vi "Compile and Export Settings.vi"(8 "error in (no error)":errorcluster, 11 "Device Item Ref in":T1 format="%.0x") -> (0 "error out":errorcluster)   [LabVIEW 2023, in "Protection and Counter Addon System Explorer.lvlib"]
uses:
  Protection and Counter Addon System Explorer.lvlib
  <vilib>/NI VeriStand/Custom Device API/Custom Device Item Ref.ctl
  Addon Shared/Types/Exported.OnCompile.ctl
  Addon Shared/Types/XNET Settings.ctl
  SubModules/Frame-Protection-Support/Source/Shared/Types/Exported Frame Settings.ctl
  SubModules/Frame-Protection-Support/Source/Shared/Types/Exported Frame Type.ctl
  SubModules/Frame-Protection-Support/Source/Shared/Types/Exported Protection Settings.ctl
  SubModules/Frame-Protection-Support/Source/Shared/Types/Protection Type.ctl
  SubModules/Frame-Protection-Support/Source/Shared/Types/XNET Signal Configuration.ctl
  SubModules/Frame-Protection-Support/Source/Shared/Types/Exported Counter Settings.ctl
  SubModules/Frame-Protection-Support/Source/Shared/Types/Exported Event Trigger Type.ctl
  Addon Shared/Types/986x.ctl
  SubModules/Frame-Protection-Support/Source/System Explorer/Types/Export Frame GUIDs List.ctl
  <vilib>/NI VeriStand/Custom Device Tools/Custom Device Utility Library/Search Direction.ctl
  SubModules/Frame-Protection-Support/Source/System Explorer/Types/Export Frames List and Type.ctl
  SubModules/Frame-Protection-Support/Source/System Explorer/Types/Exported Frame Settings.ctl
  Addon Shared/SubVIs/GUID Lookup.vi
  <vilib>/NI VeriStand/Custom Device API/NI VeriStand - Get Item Property.vi
  <vilib>/NI VeriStand/Custom Device API/Get Item Property (Boolean).vi
  <vilib>/NI VeriStand/Custom Device API/Get Item Property (String).vi
  FileDependency.Get.Target Path.vi
  <vilib>/NI VeriStand/Custom Device Tools/Custom Device Utility Library/NI VeriStand - Search for Item by GUID.vi
  <vilib>/NI VeriStand/Custom Device API/Set Item Property (Variant).vi
  <vilib>/NI VeriStand/Custom Device Tools/Custom Device Utility Library/Custom Device Utility Library.lvlib
  Addon Shared/Protection and Counter Addon Shared.lvlib
  <vilib>/NI VeriStand/Custom Device API/Custom Device API.lvlib
  SubModules/Frame-Protection-Support/Source/Shared/Protection and Counter Support Shared.lvlib
  <vilib>/NI/NIVS Inline Async API/_Data Access System Explorer/Data Access System Explorer.lvlib
  SubModules/Frame-Protection-Support/Source/System Explorer/Protection and Counter Support System Explorer.lvlib
  SubModules/Frame-Protection-Support/Source/LP_CRC/LP_CRC.lvlib
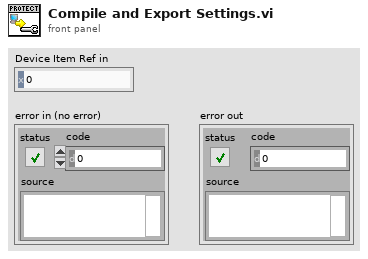
[diagram p1: front panel]
types:
  T1 = typedef "Custom Device API.lvlib/Custom Device Item Ref.ctl" = u64
  T2 = cluster{"Name":string, "Type":enum16{"Output/Write", "Input/Read", "Input/ReadWrite"}, "VS Refs":T1[]}
  T3 = typedef "Protection and Counter Support System Explorer.lvlib/Export Frames List and Type.ctl" = cluster{"Type":T4, "Frame Refs":T1[], "Frame Settings":T5[]}
  T4 = typedef "Protection and Counter Support Shared.lvlib/Exported Frame Type.ctl" = enum16{"Periodic", "Event", "Periodic/Event"}
  T5 = typedef "Protection and Counter Support System Explorer.lvlib/Exported Frame Settings.ctl" = cluster{"ID":u32, "Disable Transmission":bool, "Disable Transmission Ref":T1, "Transmit Trigger":T6, "Transmit Trigger Ref":T1, "Start Time Offset (ms)":u32}
  T6 = typedef "Protection and Counter Support Shared.lvlib/Exported Event Trigger Type.ctl" = enum16{"Channel value change", "Trigger channel (not zero)", "Channel value change or trigger channel (not zero)", "Trigger channel (any value change)", "Channel value change or trigger channel (any value change)"}
  T7 = typedef "Custom Device Utility Library.lvlib/Search Direction.ctl" = enum16{"Down", "Up"}
  T8 = typedef "Protection and Counter Support System Explorer.lvlib/Export Frame GUIDs List.ctl" = cluster{"Signal Page GUID":string, "Rolling Counter Value GUID":string, "Protection Value GUID":string, "Time Difference GUID":string, "Receive Time GUID":string}
  T9 = typedef "Protection and Counter Addon Shared.lvlib/Exported.OnCompile.ctl" = cluster{"Name":string, "XNET Settings":T10, "Frames":T11[], "986x Support":T16, "Incoming Frames":T11[], "Msg IDs":string[], "Data IDs":string[]}
  T10 = typedef "Protection and Counter Addon Shared.lvlib/XNET Settings.ctl" = cluster{"Database":refnum<k21>, "Cluster":refnum<k21>, "Port":string, "Baud rate [Bd]":u64, "Termination":u32, "CAN I/O Mode":u32, "FD Baud rate [Bd]":u64, "Priority":i32, "Use Legacy":bool, "FD ISO Mode":u32}
  T11 = typedef "Protection and Counter Support Shared.lvlib/Exported Frame Settings.ctl" = cluster{"Type":T4, "Frame ID":u32, "Payload Length":u32, "Signal XNET Paths":string[], "Frame.PrevData":dbl[], "VS Offset":i32, "VS Length":i32, "Generation Period":u32, "Has Protection?":bool, "Protection Configurations":T12[], "Has Counter":bool, "Counter Configurations":T15[], "Has Disable?":bool, "Disable VS Index":i32, "Transmit Trigger":T6, "Trigger VS Index":i32, "Start Time Offset (ms)":u32}
  T12 = typedef "Protection and Counter Support Shared.lvlib/Exported Protection Settings.ctl" = cluster{"Protection Frame Index":i32, "Protection Type":T13, "Data Indeces":i32[], "Initialized Data Array":dbl[], "Protection Signal XNET Paths":string[], "CRC Channels":T14[], "Protection VS Update Index":i32, "Override Index":i32, "Override Value Index":i32}
  T13 = typedef "Protection and Counter Support Shared.lvlib/Protection Type.ctl" = enum16{"Arb ID + Bytes Checksum with Inversion", "Arb ID + Bytes CRC with Inversion", "Reversed Raw Signal Checksum with Inversion", "Concatenated Two's Compliment", "LP_CRC8", "LP_Checksum", "LP_CRC8_MRS"}
  T14 = typedef "Protection and Counter Support Shared.lvlib/XNET Signal Configuration.ctl" = cluster{"Start Bit":i32, "Name":string, "Number of bits":i32, "Scale":dbl, "Offset":dbl, "Data Type":u32, "Counter":bool}
  T15 = typedef "Protection and Counter Support Shared.lvlib/Exported Counter Settings.ctl" = cluster{"Frame Index":i32, "Max Count":dbl, "VS Index":i32, "Bit Length":i64, "Override Index":i32, "Override Value Index":i32}
  T16 = typedef "Protection and Counter Addon Shared.lvlib/986x.ctl" = cluster{"Enable":bool, "RIO Device":string, "Bitfile":path}
  T17 = typedef "Custom Device API.lvlib/Custom Device Item Info.ctl" = cluster{"Name":string, "Is Channel":bool, "GUID":string, "Is Waveform":bool}
  T18 = typedef "Protection and Counter Addon System Explorer.lvlib/Frame Settings.ctl" = cluster{"ID":u32, "Disable Transmission":bool, "Disable Transmission Ref":T1, "Transmit Trigger":T19, "Transmit Trigger Ref":T1, "Start Time Offset (ms)":u32}
  T19 = typedef "Protection and Counter Addon System Explorer.lvlib/Event Trigger Type.ctl" = enum16{"Channel value change", "Trigger channel (not zero)", "Channel value change or trigger channel (not zero)", "Trigger channel (any value change)", "Channel value change or trigger channel (any value change)"}
  T20 = cluster{"Name":string, "Type":enum16{"Output/Write", "Input/Read", "Input/ReadWrite"}, "VS Refs":T1[]}[]
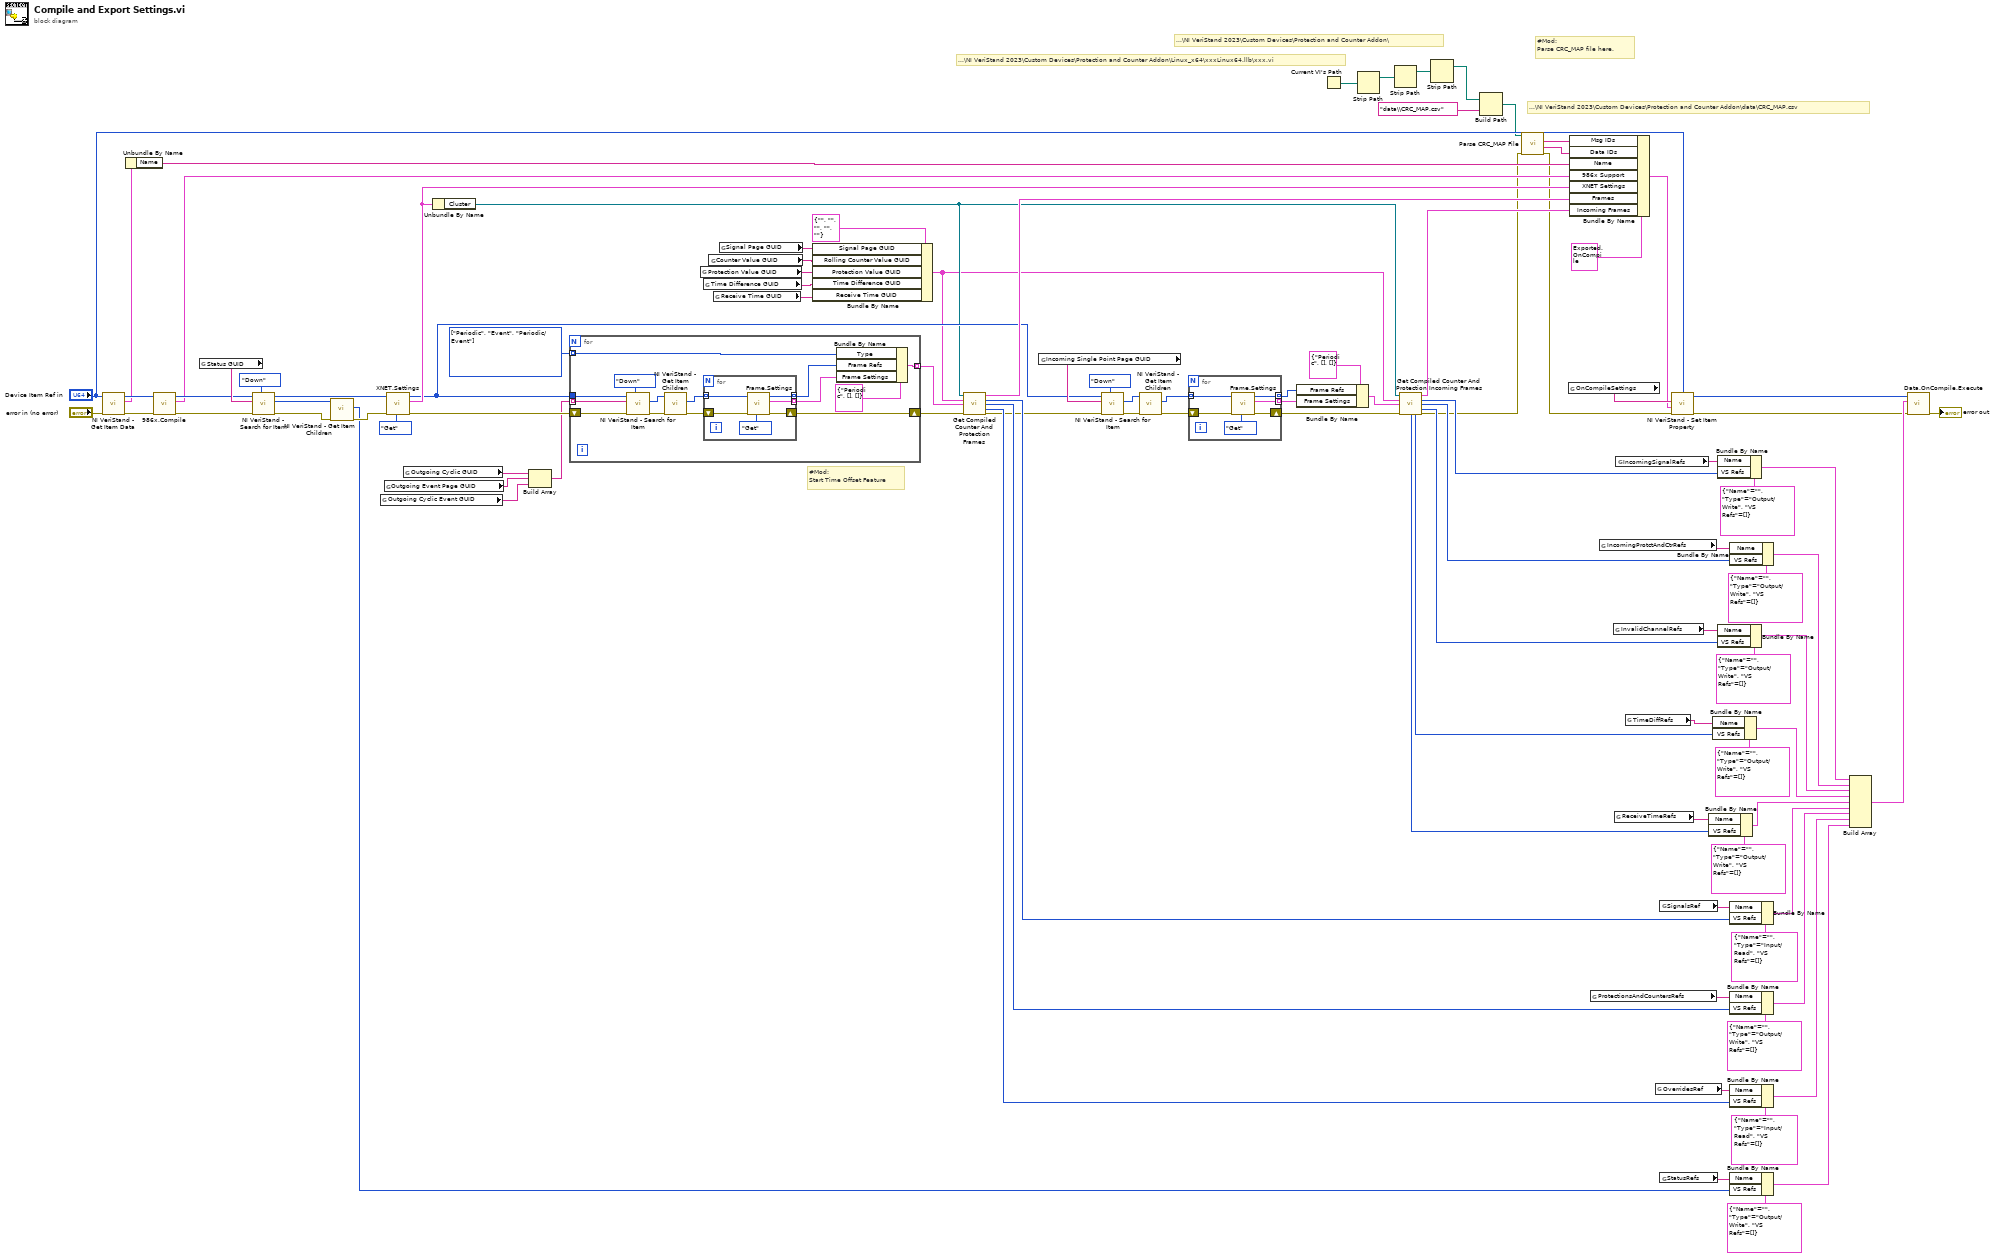
[diagram p0: block diagram]
diagram:
  w70 = T4[] [enum."Periodic", enum."Event", enum."Periodic/Event"] items=["Periodic", "Event", "Periodic/Event"]
  # "#Mod:\nParse CRC_MAP file here."
  # "...\\NI VeriStand 2023\\Custom Devices\\Protection and Counter Addon\\data\\CRC_MAP.csv"
  # "...\\NI VeriStand 2023\\Custom Devices\\Protection and Counter Addon\\"
  # "...\\NI VeriStand 2023\\Custom Devices\\Protection and Counter Addon\\Linux_x64\\xxxLinux64.llb\\xxx.vi"
  # "#Mod:\nStart Time Offset Feature"
  n1 = call <vilib>:"NI VeriStand - Get Item Data.vi"("error in (no error)"="error in (no error)", "Item Ref in"="Device Item Ref in") -> ("error out"=w57:errorcluster, "Item Info"=w55:T17, "Item Ref out"=w56:T1)  [unwired: 6 in, 1 out]
  n2 = Unbundle By Name(w55) -> ("Name"=w54:string)
  n3 = call "986x.Compile.vi"("error in (no error)"=w57, "Item Ref in"=w56) -> ("error out"=w77:errorcluster, "986x Support"=w67:T16, "Item Ref out"=w76:T1)  [unwired: 7 in]
  n4 = global read "GUID Lookup.vi" "Status GUID"() -> (w84:string)
  n5 = call-poly <vilib>:"NI VeriStand - Search for Item.vi"("Direction (Down)"=Search_Direction."Down", "error in"=w77, "Item GUID"=w84, "Section Ref in"=w76) -> ("error out"=w81:errorcluster, "Item Ref"=w82:T1, "Section Ref out"=w83:T1)  [unwired: 4 in, 1 out]
  n6 = call <vilib>:"NI VeriStand - Get Item Children.vi"("error in (no error)"=w81, "Item Ref in"=w82) -> ("error out"=w80:errorcluster, "Child Refs"=w79:T1[])  [unwired: 6 in, 2 out]
  n7 = global read "GUID Lookup.vi" "Outgoing Cyclic Event GUID"() -> (w62:string)
  n8 = global read "GUID Lookup.vi" "Outgoing Event Page GUID"() -> (w63:string)
  n9 = call "XNET.Settings.vi"("Action"=enum8{"Get", "Set"}."Get", "error in (no error)"=w80, "Parent Ref in"=w83) -> ("error out"=w61:errorcluster, "XNET Settings"=w99:T10, "Item Ref out"=w41:T1)  [unwired: 6 in]
  n10 = global read "GUID Lookup.vi" "Outgoing Cyclic GUID"() -> (w64:string)
  n11 = Unbundle By Name(w99) -> ("Cluster"=w25:refnum<k21>)
  n12 = Build Array(w64, w63, w62) -> (w60:string[])
  n13 = for {
    shift-right: [w102] -> w71
    shift-left: w61 -> [w112]
    tunnel: w70 -> [w115] mode=indexing
    tunnel: [w114] -> w69 mode=indexing
    tunnel: w41 -> [w111]
    tunnel: w60 -> [w110] mode=indexing
    n14 = call-poly <vilib>:"NI VeriStand - Search for Item.vi"("Direction (Down)"=Search_Direction."Down", "error in"=w112, "Item GUID"=w110, "Section Ref in"=w111) -> ("error out"=w108:errorcluster, "Item Ref"=w109:T1)  [unwired: 4 in, 2 out]
    n15 = call <vilib>:"NI VeriStand - Get Item Children.vi"("error in (no error)"=w108, "Item Ref in"=w109) -> ("error out"=w106:errorcluster, "Child Refs"=w105:T1[])  [unwired: 6 in, 2 out]
    n16 = for {
      tunnel: w105 -> [w119] mode=indexing
      shift-right: [w118] -> w102
      shift-left: w106 -> [w120]
      tunnel: [w117] -> w104 mode=indexing
      tunnel: [w116] -> w103 mode=indexing
      n17 = call "Frame.Settings.vi"("Action"=enum8{"Get", "Set"}."Get", "error in (no error)"=w120, "Item Ref in"=w119) -> ("error out"=w118:errorcluster, "Frame.Settings"=w116:T18, "Item Ref out"=w117:T1)  [unwired: 6 in]
    }
    n18 = Bundle By Name(cluster=T3 {"Type"=enum."Periodic", "Frame Refs"=[], "Frame Settings"=[]} ("Export Frames List and Type"), "Type"=w115, "Frame Refs"=w104, "Frame Settings"=w103) -> (w114:T3)
  }
  n19 = global read "GUID Lookup.vi" "Protection Value GUID"() -> (w73:string)
  n20 = global read "GUID Lookup.vi" "Time Difference GUID"() -> (w12:string)
  n21 = global read "GUID Lookup.vi" "Counter Value GUID"() -> (w74:string)
  n22 = global read "GUID Lookup.vi" "Receive Time GUID"() -> (w11:string)
  n23 = global read "GUID Lookup.vi" "Signal Page GUID"() -> (w75:string)
  n24 = Bundle By Name(cluster=T8 {"Signal Page GUID"="", "Rolling Counter Value GUID"="", "Protection Value GUID"="", "Time Difference GUID"="", "Receive Time GUID"=""}, "Signal Page GUID"=w75, "Rolling Counter Value GUID"=w74, "Protection Value GUID"=w73, "Time Difference GUID"=w12, "Receive Time GUID"=w11) -> (w24:T8)
  n25 = call "Get Compiled Counter And Protection Frames.vi"("XNET Cluster"=w25, "GUIDs"=w24, "Frames per type"=w69, "error in (no error)"=w71) -> ("Frames"=w65:T11[], "Signals Refs"=w66:T1[], "Counters and Protection Refs"=w94:T1[], "Override Refs"=w50:T1[], "error out"=w46:errorcluster)  [unwired: 7 in]
  n26 = global read "GUID Lookup.vi" "Incoming Single Point Page GUID"() -> (w45:string)
  n27 = call-poly <vilib>:"NI VeriStand - Search for Item.vi"("Direction (Down)"=Search_Direction."Down", "error in"=w46, "Item GUID"=w45, "Section Ref in"=w41) -> ("error out"=w47:errorcluster, "Item Ref"=w48:T1)  [unwired: 4 in, 2 out]
  n28 = call <vilib>:"NI VeriStand - Get Item Children.vi"("error in (no error)"=w47, "Item Ref in"=w48) -> ("error out"=w44:errorcluster, "Child Refs"=w42:T1[])  [unwired: 6 in, 2 out]
  n29 = for {
    tunnel: w42 -> [w125] mode=indexing
    shift-right: [w124] -> w43
    shift-left: w44 -> [w126]
    tunnel: [w123] -> w39 mode=indexing
    tunnel: [w122] -> w38 mode=indexing
    n30 = call "Frame.Settings.vi"("Action"=enum8{"Get", "Set"}."Get", "error in (no error)"=w126, "Item Ref in"=w125) -> ("error out"=w124:errorcluster, "Frame.Settings"=w122:T18, "Item Ref out"=w123:T1)  [unwired: 6 in]
  }
  n31 = Bundle By Name(cluster=T3 {"Type"=enum."Periodic", "Frame Refs"=[], "Frame Settings"=[]} ("Export Frames List and Type"), "Frame Refs"=w39, "Frame Settings"=w38) -> (w23:T3)
  n32 = Current VI's Path() -> (path=w10:path)
  n33 = Strip Path(path=w10) -> (stripped path=w9:path)  [unwired: 1 out]
  n34 = Strip Path(path=w9) -> (stripped path=w8:path)  [unwired: 1 out]
  n35 = call "Get Compiled Counter And Protection Incoming Frames.vi"("XNET Cluster"=w25, "GUIDs"=w24, "Incoming Frames In"=w23, "error in (no error)"=w43) -> ("Incoming Frames Out"=w22:T11[], "Signals Refs"=w21:T1[], "Counters and Protection Refs"=w20:T1[], "Invalid Refs"=w19:T1[], "Rcv Time Refs"=w17:T1[], "Time Diff Refs"=w18:T1[], "error out"=w2:errorcluster)  [unwired: 5 in]
  n36 = Strip Path(path=w8) -> (stripped path=w7:path)  [unwired: 1 out]
  n37 = Build Path(base path=w7, name or relative path="data\\CRC_MAP.csv") -> (appended path=w3:path)
  n38 = call "Parse CRC_MAP File.vi"("error in"=w2, "file (use dialog)"=w3) -> ("error out"=w1:errorcluster, "Data IDs"=w4:string[], "Msg IDs"=w5:string[])  [unwired: 6 in, 1 out]
  n39 = global read "GUID Lookup.vi" "OnCompileSettings"() -> (w89:string)
  n40 = Bundle By Name(cluster=T9 {"Name"="", "XNET Settings"={"Database"="", "Cluster"="", "Port"="", "Baud rate [Bd]"=500000, "Termination"=1, "CAN I/O Mode"=0, "FD Baud rate [Bd]"=500000, "Priority"=100, "Use Legacy"=FALSE, "FD ISO Mode"=0}, "Frames"=[], "986x Support"={"Enable"=FALSE, "RIO Device"="", "Bitfile"=path ""}, "Incoming Frames"=[], "Msg IDs"=[], "Data IDs"=[]}, "Msg IDs"=w5, "Data IDs"=w4, "Name"=w54, "986x Support"=w67, "XNET Settings"=w99, "Frames"=w65, "Incoming Frames"=w22) -> (w30:T9)
  n41 = global read "GUID Lookup.vi" "ProtectionsAndCountersRefs"() -> (w90:string)
  n42 = global read "GUID Lookup.vi" "IncomingProtctAndCtrRefs"() -> (w26:string)
  n43 = global read "GUID Lookup.vi" "InvalidChannelRefs"() -> (w34:string)
  n44 = global read "GUID Lookup.vi" "ReceiveTimeRefs"() -> (w33:string)
  n45 = global read "GUID Lookup.vi" "IncomingSignalRefs"() -> (w35:string)
  n46 = global read "GUID Lookup.vi" "TimeDiffRefs"() -> (w29:string)
  n47 = global read "GUID Lookup.vi" "OverridesRef"() -> (w53:string)
  n48 = global read "GUID Lookup.vi" "SignalsRef"() -> (w91:string)
  n49 = global read "GUID Lookup.vi" "StatusRefs"() -> (w86:string)
  n50 = call-poly <vilib>:"NI VeriStand - Set Item Property.vi"("error in (no error)"=w1, "Value"=w30, "Property Name"=w89, "Item Ref in"="Device Item Ref in") -> ("error out"=w93:errorcluster, "Item Ref out"=w92:T1)  [unwired: 5 in, 1 out]
  n51 = Bundle By Name(cluster=T2 {"Name"="", "Type"=enum."Output/Write", "VS Refs"=[]} ("Group"), "Name"=w33, "VS Refs"=w17) -> (w13:T2)
  n52 = Bundle By Name(cluster=T2 {"Name"="", "Type"=enum."Output/Write", "VS Refs"=[]} ("Group"), "Name"=w29, "VS Refs"=w18) -> (w14:T2)
  n53 = Bundle By Name(cluster=T2 {"Name"="", "Type"=enum."Output/Write", "VS Refs"=[]} ("Group"), "Name"=w35, "VS Refs"=w21) -> (w31:T2)
  n54 = Bundle By Name(cluster=T2 {"Name"="", "Type"=enum."Output/Write", "VS Refs"=[]} ("Group"), "Name"=w34, "VS Refs"=w19) -> (w15:T2)
  n55 = Bundle By Name(cluster=T2 {"Name"="", "Type"=enum."Input/Read", "VS Refs"=[]} ("Group"), "Name"=w91, "VS Refs"=w66) -> (w97:T2)
  n56 = Bundle By Name(cluster=T2 {"Name"="", "Type"=enum."Output/Write", "VS Refs"=[]} ("Group"), "Name"=w90, "VS Refs"=w94) -> (w88:T2)
  n57 = Bundle By Name(cluster=T2 {"Name"="", "Type"=enum."Input/Read", "VS Refs"=[]} ("Group"), "Name"=w53, "VS Refs"=w50) -> (w51:T2)
  n58 = Bundle By Name(cluster=T2 {"Name"="", "Type"=enum."Output/Write", "VS Refs"=[]} ("Group"), "Name"=w86, "VS Refs"=w79) -> (w68:T2)
  n59 = Bundle By Name(cluster=T2 {"Name"="", "Type"=enum."Output/Write", "VS Refs"=[]} ("Group"), "Name"=w26, "VS Refs"=w20) -> (w16:T2)
  n60 = Build Array(w31, w16, w15, w14, w13, w97, w88, w51, w68) -> (w96:T20)
  n61 = call <vilib>:"Data.OnCompile.Execute.vi"("error in"=w93, "VS Ref Groups"=w96, "Custom Device Ref"=w92) -> ("error out"=→"error out":errorcluster)  [unwired: 7 in, 1 out]
